vi "Set Shutter Ex.vi"(6 "extmode":i32, 7 "openingtime":i32, 8 "error in (no error)":errorcluster, 9 "closingtime":i32, 10 "mode":i32, 11 "typ":i32) -> (0 "error out":errorcluster, 3 "function return":u32)   [LabVIEW 2014, in "atmcd32d.lvlib"]
doc: "unsigned int WINAPI SetShutterEx(int typ, int mode, int closingtime, int openingtime, int extmode);"
uses:
  atmcd32d.lvlib
  atmcd32d.dll
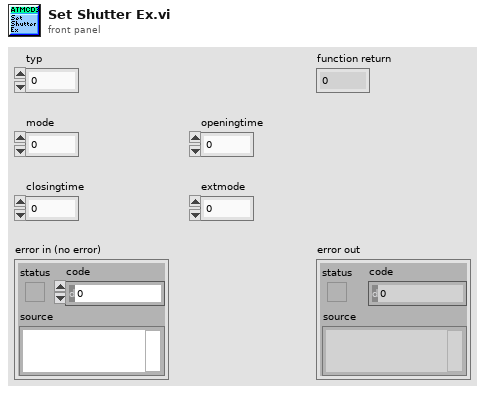
[diagram p1: front panel]
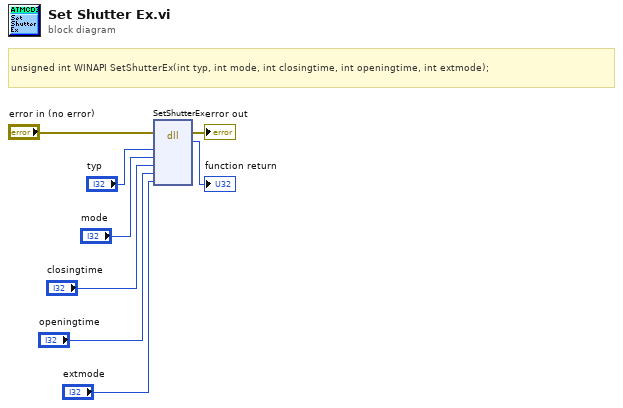
[diagram p0: block diagram]
diagram:
  # "unsigned int WINAPI SetShutterEx(int typ, int mode, int closingtime, int openingtime, int extmode);"
  n1 = dll-call lib="C:/Users/Bakir/Documents/Lambda2-Testing/lib/Andorlib/atmcd32d.*" fn="SetShutterEx"(error in="error in (no error)", "typ"="typ", "mode"="mode", "closingtime"="closingtime", "openingtime"="openingtime", "extmode"="extmode") -> (error out=→"error out":errorcluster, →"function return":u32)  [unwired: 7 in, 1 out]
